vi "AO Sample.vi"() -> ()   [LabVIEW 2016]
uses:
  <vilib>/DAQmx/write.llb/DAQmx Write (Analog 1D Wfm NChan NSamp).vi
  <vilib>/DAQmx/create/channels.llb/DAQmx Create Channel (AO-Voltage-Basic).vi
  <vilib>/DAQmx/configure/timing.llb/DAQmx Timing (Sample Clock).vi
  <vilib>/DAQmx/miscellaneous.llb/DAQmx Fill In Error Info.vi
  <resource>/objmgr/daqmx.rc
  <vilib>/measure/NI_MABase.lvlib
panel:
  in  "Noise Amplitude":dbl=1.0 format="%#_13g"
  in  "Waveform":T1={"Waveform Type"=0, "Amplitude"=1, "Freqency"=300.0} {"Waveform Type" items=["正弦波", "三角波", "方形波", "ノコギリ波"]}
  out "Output Signal":waveform(dbl)[](graph)=[{"t0"=timestamp(0 s since 1904-01-01), "dt"=2e-05, "Y"=array[5000 elements]}, {"t0"=timestamp(0.10000000000000002 s since 1904-01-01), "dt"=2e-05, "Y"=array[5000 elements]}]
  in  "Number of Sample":i32=5000
  in  "Sample Rate":dbl=50000.0
  in  "Sample Clock Source":tag="OnboardClock"
  in  "MaxVoltage":dbl=5.0
  in  "MinVoltage":dbl=-5.0
  in  "PhyicalChannel":tag="cDAQ2Mod3/ao0:1"
  out "Actual Sampling Rate":dbl=50000.0 format="%0.2f"
  in  "一時停止":bool
  # "ao0 is Reference signal\nao1 is simulated noisy signal went through DUT for debug.\nIf you do not have DUT, please use ao1."
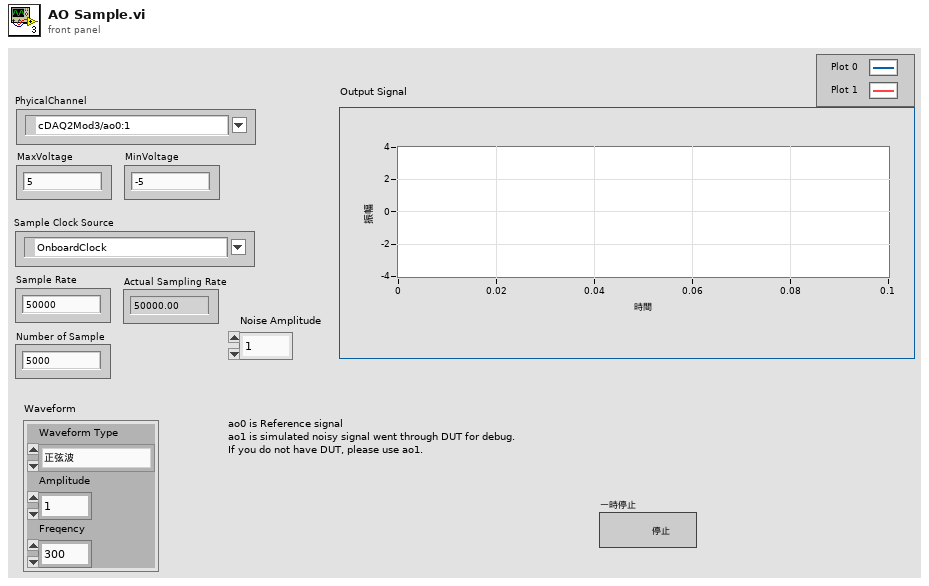
[diagram p1: front panel]
types:
  T1 = cluster{"Waveform Type":u16, "Amplitude":i32, "Freqency":dbl}
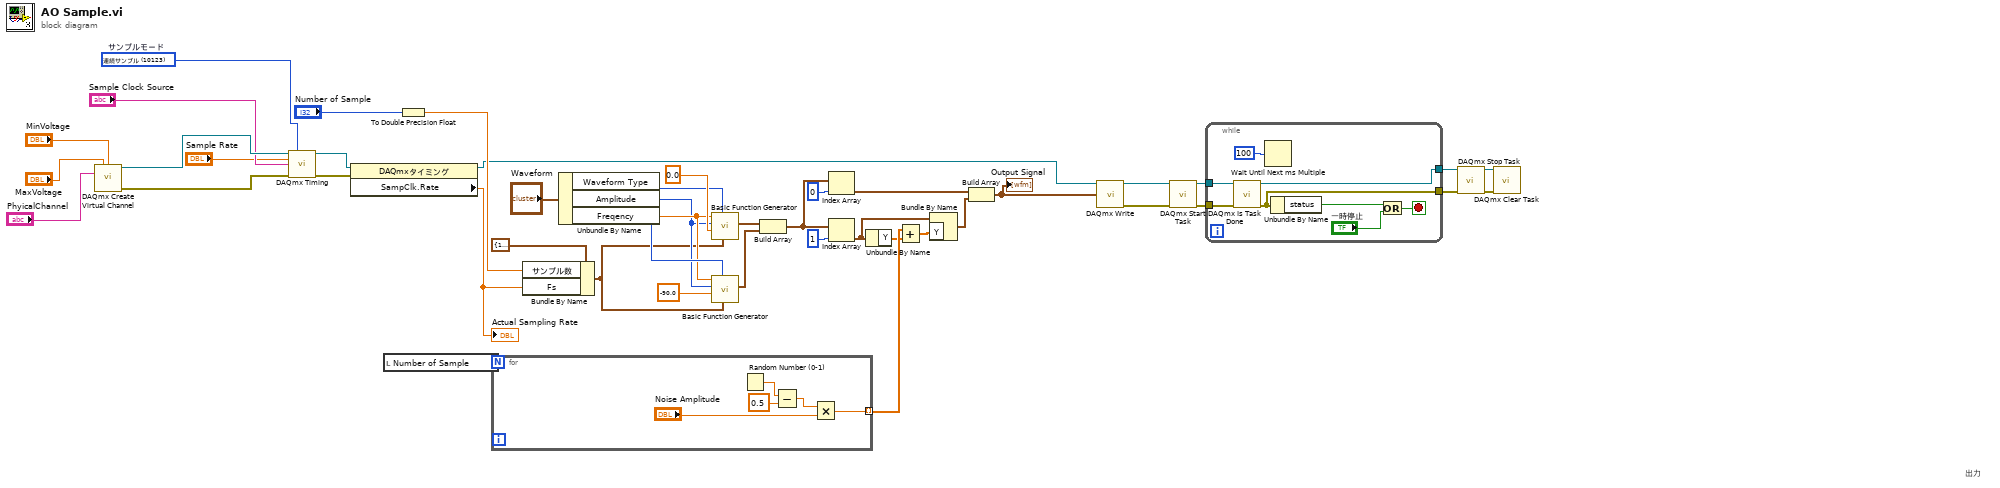
[diagram p0: block diagram]
diagram:
  w41 = 10123 items=["有限サンプル"=10178, "連続サンプル"=10123, "ハードウェアタイミングシングルポイント"=12522]  # サンプルモード
  # "出力"
  n1 = call-poly <vilib>:"DAQmx Create Virtual Channel.vi"("maximum value"="MaxVoltage", "minimum value"="MinVoltage", "physical channels"="PhyicalChannel") -> ("task out"=w39:refnum<k21>, "error out"=w40:errorcluster)  [unwired: 11 in]
  n2 = call-poly <vilib>:"DAQmx Timing.vi"("task/channels in"=w39, "sample mode"=w41, "rate"="Sample Rate", "source"="Sample Clock Source", "error in"=w40) -> ("task out"=w43:refnum<k21>, "error out"=w42:errorcluster)  [unwired: 9 in]
  n3 = property class="DAQmxタイミング"(reference=w43, error in=w42) -> (reference out=w25:refnum<k21>, "SampClk.Rate"=w30:dbl)  [unwired: 1 out]
  "Actual Sampling Rate" <- w30
  n4 = local read "Number of Sample"() -> (w22:i32)
  n5 = To Double Precision Float(number="Number of Sample") -> (double precision float=w27:dbl)
  n6 = for {
    N: w22 -> [_]
    tunnel: [w44] -> w21 mode=indexing
    n7 = Random Number (0-1)() -> (number: 0 to 1=w48:dbl)
    n8 = Subtract(x=w48, y=0.5) -> (x-y=w46:dbl)
    n9 = Multiply(x=w46, y="Noise Amplitude") -> (x*y=w44:dbl)
  }
  n10 = Bundle By Name(cluster=cluster{"Fs":dbl, "サンプル数":dbl} {"Fs"=1000.0, "サンプル数"=1000.0} ("サンプリング情報"), "サンプル数"=w27, "Fs"=w30) -> (w3:cluster{"Fs":dbl, "サンプル数":dbl})
  n11 = Unbundle By Name("Waveform") -> ("Waveform Type"=w10:u16, "Amplitude"=w8:i32, "Freqency"=w9:dbl)
  n12 = call <vilib>:"Basic Function Generator.vi"("sampling info"=w3, "signal type"=w10, "phase"=0.0, "amplitude"=w8, "frequency"=w9) -> ("signal out"=w6:waveform(dbl))  [unwired: 4 in, 2 out]
  n13 = call <vilib>:"Basic Function Generator.vi"("sampling info"=w3, "signal type"=w10, "phase"=-90.0, "amplitude"=w8, "frequency"=w9) -> ("signal out"=w5:waveform(dbl))  [unwired: 4 in, 2 out]
  n14 = Build Array(w6, w5) -> (w4:waveform(dbl)[])
  n15 = Index Array(array=w4, index=0 ("指標")) -> (element=w17:waveform(dbl))
  n16 = Index Array(array=w4, index=1 ("指標")) -> (element=w19:waveform(dbl))
  n17 = Unbundle By Name(w19) -> ("Y"=w20:dbl[])
  n18 = Add(x=w21, y=w20) -> (x+y=w18:dbl[])
  n19 = Bundle By Name(cluster=w19, "Y"=w18) -> (w16:waveform(dbl))
  n20 = Build Array(w17, w16) -> (w15:waveform(dbl)[])
  "Output Signal" <- w15
  n21 = call-poly <vilib>:"DAQmx Write.vi"("task/channels in"=w25, "data"=w15) -> ("task out"=w29:refnum<k21>, "error out"=w28:errorcluster)  [unwired: 11 in, 1 out]
  n22 = call <vilib>:"DAQmx Start Task.vi"("task/channels in"=w29, "error in"=w28) -> ("task out"=w38:refnum<k21>, "error out"=w37:errorcluster)  [unwired: 12 in]
  n23 = while {
    tunnel: w38 -> [w56]
    tunnel: w37 -> [w55]
    tunnel: [w52] -> w13
    tunnel: [w53] -> w14
    stop <- w54 stop-if-true
    n24 = call <vilib>:"DAQmx Is Task Done.vi"("task/channels in"=w56, "error in"=w55) -> ("task out"=w53:refnum<k21>, "error out"=w52:errorcluster)  [unwired: 11 in, 1 out]
    n25 = Wait Until Next ms Multiple(millisecond multiple=u32 100 ("ミリ秒倍数")) -> ()  [unwired: 1 out]
    n26 = Unbundle By Name(w52) -> ("status"=w51:bool)
    n27 = Or(x=w51, y="一時停止") -> (x .or. y?=w54:bool)
  }
  n28 = call <vilib>:"DAQmx Stop Task.vi"("task/channels in"=w14, "error in"=w13) -> ("task out"=w1:refnum<k21>, "error out"=w2:errorcluster)  [unwired: 12 in]
  n29 = call <vilib>:"DAQmx Clear Task.vi"("task in"=w1, "error in"=w2) -> ()  [unwired: 13 in, 1 out]
